vi "PH_USB600x_AnalogReader.PC Set Prdc Interval.vi"(0 "i ref in":refnum<vi>, 2 "prdc interval [s]":dbl, 5 "error IO":errorcluster) -> (14 "i ref out":refnum<vi>, 19 "error out":errorcluster)   [LabVIEW 2014, in "PH_USB600x_AnalogReader.lvlib"]
uses:
  PH_USB600x_AnalogReader.lvlib
  PH_Basics/PH_Common/PH_Common.lvlib
  CS_Core/BaseProcess/BaseProcess.lvlib
  CS_Core/CSSystem/CSSystemLib/CSSystemLib.lvlib
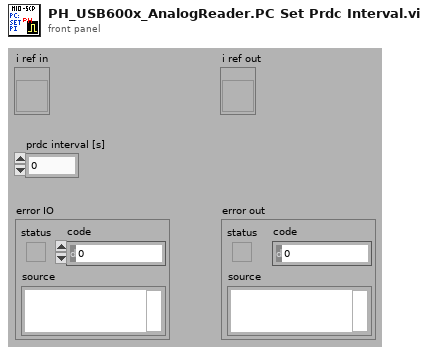
[diagram p1: front panel]
types:
  T1 = enum16{"simple", "synchronous", "asynchronous", "notification"}
  T2 = typedef "PH_USB600x_AnalogReader.lvlib/PH_USB600x_AnalogReader.i attribute.ctl" = cluster{"GUI Refs":cluster{"Delete":refnum<vi>, "Status":refnum<vi>, "Timeout":refnum<vi>, "Acquire Waveform":refnum<vi>, "Timing":refnum<vi>, "Graph":refnum<vi>, "Prdc Interval":refnum<vi>, "Formula":refnum<vi>}, "Device Settings":cluster{"AIChannel":refnum<k21>, "channelName":string, "Status":T3}, "Timing":T4, "Prdc Interval":dbl, "Lin Scaling":T5, "Data":cluster{"t0":timestamp, dbl}[]}
  T3 = typedef "PH_StatusHandler.lvlib/PH_StatusHandler.Status.ctl" = i16
  T4 = typedef "PH_USB600x_AnalogReader.lvlib/PH_USB600x_AnalogReader.Timing.ctl" = cluster{"Samples per Channel":i32, "Rate":dbl}
  T5 = typedef "PH_USB600x_AnalogReader.lvlib/PH_USB600x_AnalogReader.Lin Scaling.ctl" = cluster{"Slope [Unit/V]":dbl, "Offset [Unit]":dbl, "Y-Unit":string, "Y-Label":string}
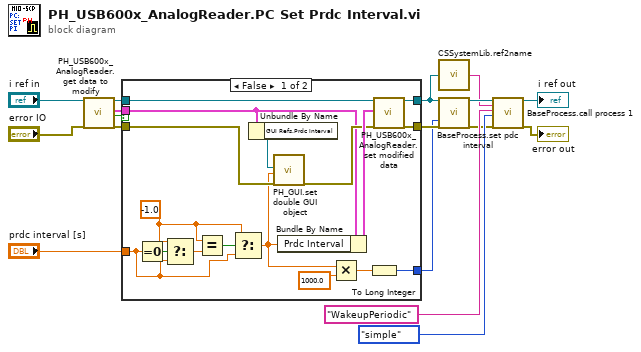
[diagram p0: block diagram]
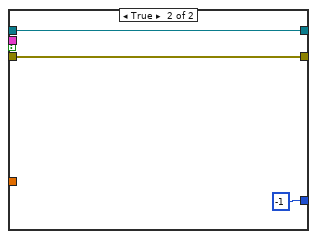
[diagram p2: hidden frame]
diagram:
  n1 = call "PH_USB600x_AnalogReader.get data to modify.vi"("i ref in"="i ref in", "error in (no error)"="error IO") -> ("i ref out"=w1:refnum<vi>, "i attribute"=w6:T2, "timed out"=w5:bool, "error out"=w2:errorcluster)  [unwired: 14 in]
  n2 = case shown="False" w5 {
    tunnel: w1 -> [w34 w37]
    tunnel: w2 -> [w30 w36]
    tunnel: [w33 w36] -> w15
    tunnel: [w32 w37] -> w17
    tunnel: w6 -> [w28 _]
    tunnel: "prdc interval [s]" -> [w20 _]
    tunnel: [w21 -1] -> w12
    frame False {
      w22 = -1.0 ("y")
      n3 = Equal To 0?(x=w20) -> (x = 0?=w25:bool)
      n4 = Select(t=w22, s=w25, f=w20) -> (s? t:f=w24:dbl)
      n5 = Equal?(x=w22, y=w24) -> (x = y?=w23:bool)
      n6 = Select(t=w22, s=w23, f=w20) -> (s? t:f=w19:dbl)
      n7 = Unbundle By Name(w28) -> ("GUI Refs.Prdc Interval"=w27:refnum<vi>)
      n8 = call "PH_GUI.set double GUI object.vi"("GUI object Ref"=w27, "value"=w19, "error in (no error)"=w30) -> ("error out"=w29:errorcluster)  [unwired: 16 in]
      n9 = Bundle By Name(cluster=w28, "Prdc Interval"=w19) -> (w31:T2)
      n10 = Multiply(x=w19, y=1000.0) -> (x*y=w18:dbl)
      n11 = To Long Integer(number=w18) -> (32bit integer=w21:i32)
      n12 = call "PH_USB600x_AnalogReader.set modified data.vi"("i ref in"=w34, "i attribute"=w31, "error in (no error)"=w29) -> ("i ref out"=w32:refnum<vi>, "error out"=w33:errorcluster)  [unwired: 15 in]
    }
    frame True {
    }
  }
  n13 = call "CSSystemLib.ref2name.vi"("obj refnum"=w17) -> ("name"=w10:string)
  n14 = call "BaseProcess.set pdc interval.vi"("i ref in"=w17, "PeriodicInterval [ms]"=w12, "error in (no error)"=w15) -> ("i ref out"=w16:refnum<vi>, "error out"=w8:errorcluster)  [unwired: 14 in, 1 out]
  n15 = call "BaseProcess.call process 1.vi"("i ref in"=w16, "Object"=w10, "Selector"="WakeupPeriodic", "CallType"=T1."simple", "error in (no error)"=w8) -> ("i ref out"=→"i ref out":refnum<vi>, "error out"=→"error out":errorcluster)  [unwired: 12 in, 1 out]
